vi "DF PROFINET IO GettingStarted Device.vi"() -> ()   [LabVIEW 2019]
doc: "This VI shows how output and input bytes can be read and write from and to a Slot of the KUNBUS DF PROFINET IO interface card as Device."
uses:
  <vilib>/KUNBUS GmbH/DF PROFINET IO/CS_PN_Device_StartStopMode.ctl
  <vilib>/Utility/error.llb/DialogType.ctl
panel:
  in  "Update time (ms)":u32=1
  in  "Tab Control":enum32{"Cyclic IO-Data"}(tab)
  in  "Slot":i32=1 caption="(-1: AllSlots)"
  in  "Get APDU status desc":bool
  out "Description:":string
  out "APDU status":u8 format="%.0x"
  out "Output data:":string
  out "Output status 3":bool
  out "Output status":u8 format="0x%02x"
  out "Input data:":string
  out "Input status 2":bool
  out "Input status":u8 format="0x%02x"
  in  "Modify input data:":string
  in  "Set input data":bool
  in  "Input status":bool=TRUE caption="Status"
  out "APDU status:":bool
  in  "Slot1: CMD":bool[][](array[boolean])
  out "Slot3: Alarm":bool[][](array[boolean])
  out "Slot4: Alarm/Status":bool[][](array[boolean])
  out "Slot5: alanog Signal":sgl[](array[numeric])
  in  "Number of Elements":i32=22
  out "Input data":u8[](array[numeric])
  out "Slot6: alanog H-L":sgl[](array[numeric])
  in  "Number of Elements":i32=22
  in  "PROFINET Device":refnum<visa-resource-name>
  in  "Stop":bool
  # "Instructions:\n1. Read the Getting Started manual: Help >> KUNBUS GmbH >> DF PROFINET IO\n2. Choose the DF PROFINET IO interface card from the VISA control \"PROFINET Device\" and then start the VI"
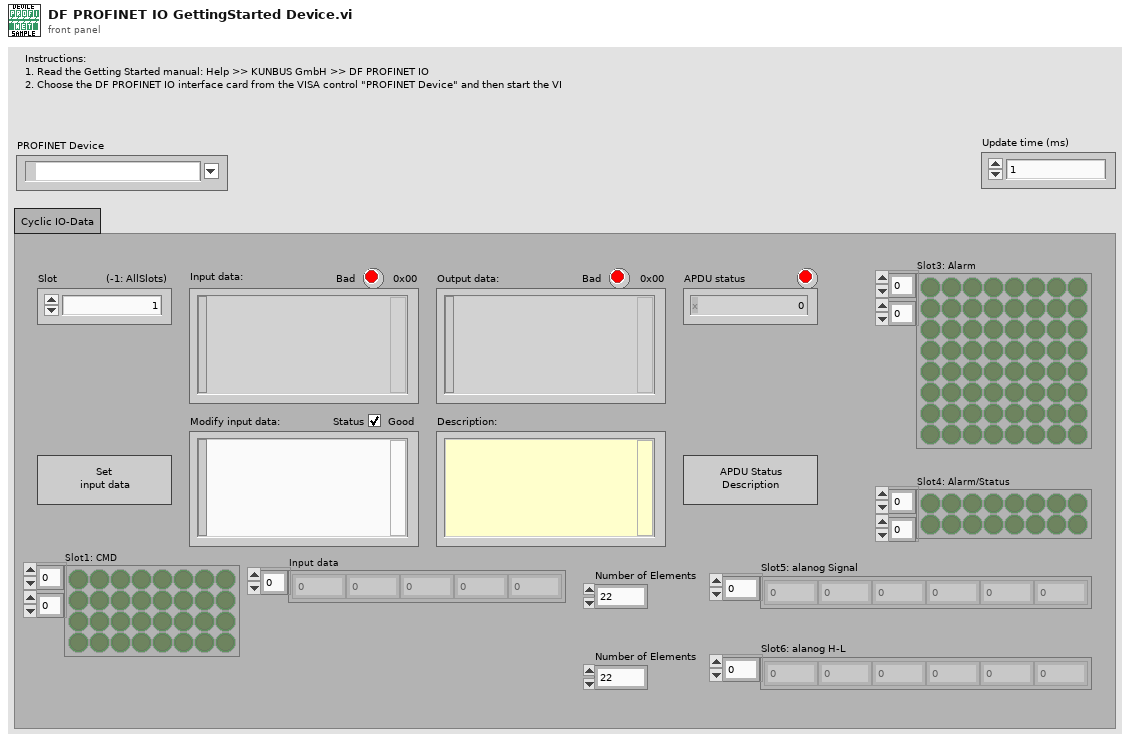
[diagram p1: front panel]
types:
  T1 = typedef "CS_PN_Device_StartStopMode.ctl" = enum32{"Start Device", "Stop Device"}
  T2 = cluster{"Slot":i32, "Output status":u8, "unsigned byte array":u8[]}[]
  T3 = cluster{"APDU status":u8, "Device status":u8, "Input status":u8, "Input data":u8[], "Output status":u8, "Output data":u8[]}
  T4 = cluster{"APDU status":u8, "Device status":u8, "Input status":u8, "Input data":u8[], "Output status":u8, "Output data":u8[]}[]
  T5 = typedef "DialogType.ctl" = u16
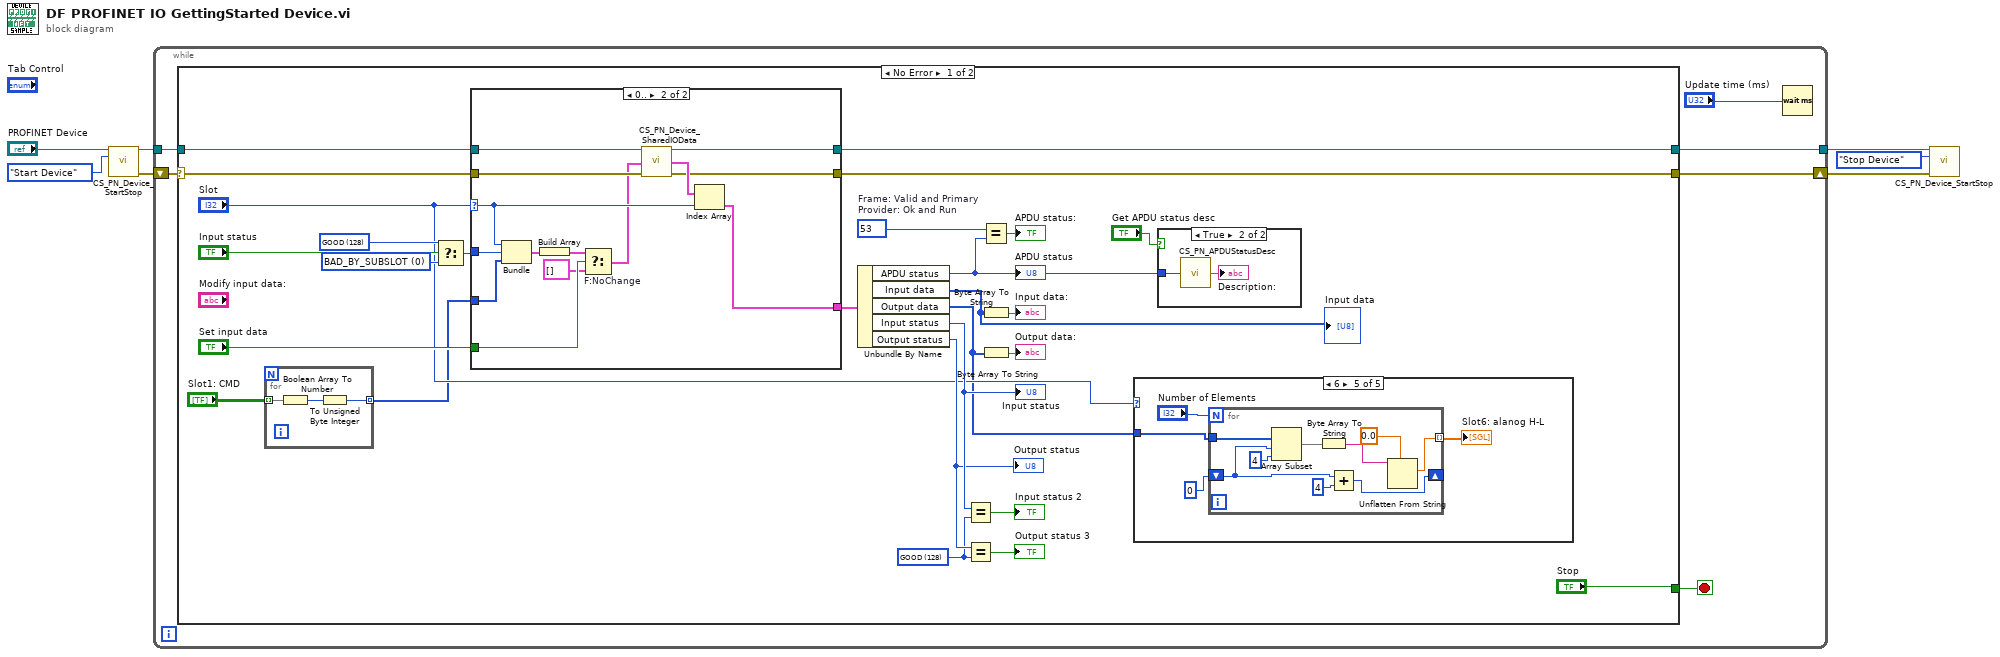
[diagram p0: block diagram]
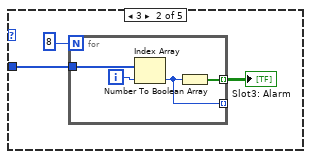
[diagram p3: hidden frame]
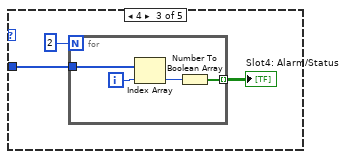
[diagram p4: hidden frame]
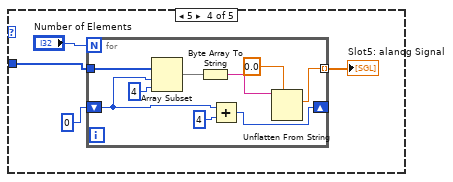
[diagram p5: hidden frame]
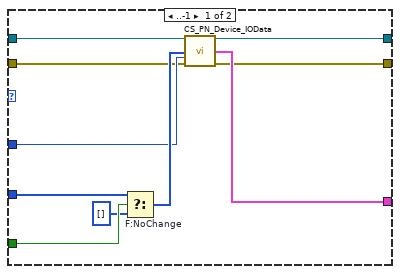
[diagram p6: hidden frame]
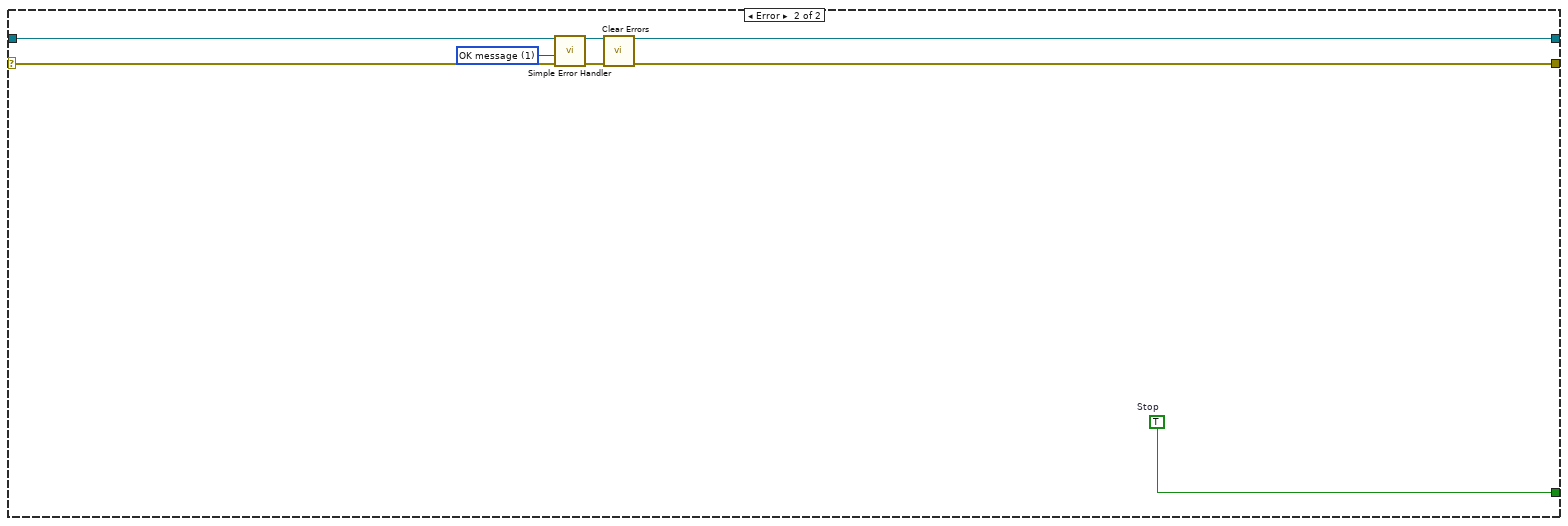
[diagram p8: hidden frame]
diagram:
  n1 = call <vilib>:"CS_PN_Device_StartStop.vi"("PN-Device resource name"="PROFINET Device", "Mode"=CS_PN_Device_StartStopMode."Start Device") -> ("PN-Device resource name out"=w3:refnum<visa-resource-name>, "Error Out"=w2:errorcluster)  [unwired: 11 in, 1 out]
  n2 = while {
    tunnel: w3 -> [w12]
    tunnel: [w11] -> w7
    shift-right: [w10] -> w4
    shift-left: w2 -> [w9]
    stop <- w8 stop-if-true
    n3 = case shown="No Error" w9 {
      selector: w9 -> [w21 w111]
      tunnel: w12 -> [w37 w114]
      tunnel: [w36 w114] -> w11
      tunnel: [w35 w115] -> w10
      tunnel: ["Stop" w110] -> w8
      frame No Error {
        w20 = u8 128 items=["BAD"=0, "GOOD"=128] ("Output status")
        w24 = u8 128 items=["BAD"=0, "GOOD"=128] ("Output status")
        w25 = u8 0 items=["BAD_BY_SUBSLOT"=0, "BAD_BY_SLOT"=32, "BAD_BY_DEVICE"=64, "BAD_BY_CONTROLLER"=96, "GOOD"=128] ("Output status")
        w31 = u8 53  # Frame: Valid and Primary Provider: Ok and Run
        n4 = for {
          tunnel: "Slot1: CMD" -> [w83] mode=indexing
          tunnel: [w81] -> w14 mode=indexing
          n5 = Boolean Array To Number(Boolean array=w83) -> (number=w82:u32)
          n6 = To Unsigned Byte Integer(number=w82) -> (unsigned 8bit integer=w81:u8)
        }
        n7 = Select(t=w24, s="Input status", f=w25) -> (s? t:f=w22:u8)
        n8 = case shown="0.." "Slot" {
          selector: "Slot" -> [_ w95]
          tunnel: w21 -> [w86 w106]
          tunnel: w37 -> [w91 w105]
          tunnel: [w90 w104] -> w36
          tunnel: [w89 w103] -> w35
          tunnel: [w92 w102] -> w27
          tunnel: "Set input data" -> [w85 w98]
          tunnel: w22 -> [w88 w100]
          tunnel: w14 -> [w87 w99]
          frame ..-1 {
            n9 = Select "F:NoChange"(t=w87, s=w85, f=u8[] []) -> (s? t:f=w93:u8[])
            n10 = call <vilib>:"CS_PN_Device_IOData.vi"("PN-Device resource name"=w91, "Input data"=w93, "Input status"=w88, "Error In"=w86) -> ("PN-Device resource name out"=w90:refnum<visa-resource-name>, "Device data"=w92:T3, "Error Out"=w89:errorcluster)  [unwired: 8 in, 1 out]
          }
          frame 0.. {
            n11 = Bundle("Slot"=w95, "Output status"=w100, w99) -> (w101:cluster{"Slot":i32, "Output status":u8, u8[]})  [unwired: 1 in]
            n12 = Build Array(w101) -> (w97:cluster{"Slot":i32, "Output status":u8, u8[]}[])
            n13 = Select "F:NoChange"(t=w97, s=w98, f=T2 []) -> (s? t:f=w94:T2)
            n14 = call <vilib>:"CS_PN_Device_SharedIOData.vi"("PN-Device resource name"=w105, "Input data"=w94, "Error In"=w106) -> ("PN-Device resource name out"=w104:refnum<visa-resource-name>, "Device data"=w107:T4, "Error Out"=w103:errorcluster)  [unwired: 9 in, 1 out]
            n15 = Index Array(array=w107, index=w95) -> (element=w102:T3)
          }
        }
        n16 = Unbundle By Name(w27) -> ("APDU status"=w29:u8, "Input data"=w32:u8[], "Output data"=w15:u8[], "Input status"=w40:u8, "Output status"=w33:u8)
        "Input status" <- w40
        "Output status" <- w33
        "APDU status" <- w29
        "Input data" <- w32
        n17 = Equal?(x=w40, y=w20) -> (x = y?=→"Input status 2":bool)
        n18 = Equal?(x=w33, y=w20) -> (x = y?=→"Output status 3":bool)
        n19 = Equal?(x=w31, y=w29) -> (x = y?=→"APDU status:":bool)
        n20 = Byte Array To String(unsigned byte array=w32) -> (string=→"Input data:":string)
        n21 = Byte Array To String(unsigned byte array=w15) -> (string=→"Output data:":string)
        n22 = case shown="6" "Slot" {
          tunnel: w15 -> [_ w41 w48 w56 w69]
          frame 0, Default {
          }
          frame 3 {
            n23 = for {
              N: 8 -> [_]
              tunnel: w41 -> [w47]
              tunnel: [w45] -> w43 mode=indexing
              tunnel: [w44] -> _ mode=indexing
              i -> [w46]
              n24 = Index Array(array=w47, index=w46) -> (element=w44:u8)
              n25 = Number To Boolean Array(number=w44) -> (Boolean array=w45:bool[])
            }
            "Slot3: Alarm" <- w43
          }
          frame 4 {
            n26 = for {
              N: 2 -> [_]
              tunnel: w48 -> [w54]
              tunnel: [w52] -> w50 mode=indexing
              i -> [w53]
              n27 = Index Array(array=w54, index=w53) -> (element=w51:u8)
              n28 = Number To Boolean Array(number=w51) -> (Boolean array=w52:bool[])
            }
            "Slot4: Alarm/Status" <- w50
          }
          frame 5 {
            n29 = for {
              N: "Number of Elements" -> [_]
              tunnel: w56 -> [w62]
              shift-right: [w60] -> _
              shift-left: 0 ("index") -> [w61]
              tunnel: [w59] -> w55 mode=indexing
              n30 = Array Subset(array=w62, index=w61, length=4) -> (w65:u8[])
              n31 = Byte Array To String(unsigned byte array=w65) -> (string=w66:string)
              n32 = Add(x=w61, y=4) -> (x+y=w60:i32)
              n33 = Unflatten From String(type=sgl 0.0 ("Data-4 byte single"), binary string=w66) -> (value=w59:sgl)  [unwired: 3 in, 2 out]
            }
            "Slot5: alanog Signal" <- w55
          }
          frame 6 {
            n34 = for {
              N: "Number of Elements" -> [_]
              tunnel: w69 -> [w75]
              shift-right: [w73] -> _
              shift-left: 0 ("index") -> [w74]
              tunnel: [w72] -> w68 mode=indexing
              n35 = Array Subset(array=w75, index=w74, length=4) -> (w78:u8[])
              n36 = Byte Array To String(unsigned byte array=w78) -> (string=w79:string)
              n37 = Add(x=w74, y=4) -> (x+y=w73:i32)
              n38 = Unflatten From String(type=sgl 0.0 ("Data-4 byte single"), binary string=w79) -> (value=w72:sgl)  [unwired: 3 in, 2 out]
            }
            "Slot6: alanog H-L" <- w68
          }
        }
        n39 = case shown="True" "Get APDU status desc" {
          tunnel: w29 -> [_ w109]
          frame False {
          }
          frame True {
            n40 = call <vilib>:"CS_PN_APDUStatusDesc.vi"("APDU Status"=w109) -> ("Description:"=→"Description:":string)  [unwired: 14 in]
          }
        }
      }
      frame Error {
        w110 = TRUE  # Stop
        w113 = T5 1 items=["no dialog", "OK message", "continue or stop message", "OK message + warnings", "continue/stop + warnings"] ("type of dialog (OK msg:1)")
        n41 = call <vilib>:"Simple Error Handler.vi"("type of dialog (OK msg:1)"=w113, "error in (no error)"=w111) -> ("error out"=w112:errorcluster)  [unwired: 3 in, 4 out]
        n42 = call <vilib>:"Clear Errors.vi"("error in (no error)"=w112) -> ("error out"=w115:errorcluster)  [unwired: 5 in, 1 out]
      }
    }
    n43 = Wait (ms)(milliseconds to wait="Update time (ms)") -> ()  [unwired: 1 out]
  }
  n44 = call <vilib>:"CS_PN_Device_StartStop.vi"("PN-Device resource name"=w7, "Mode"=CS_PN_Device_StartStopMode."Stop Device", "Error In"=w4) -> ()  [unwired: 10 in, 3 out]
